vi "Constructor.vi"(7 "TimeZoneInfoId":string, 8 "error in":errorcluster, 9 "ProductFullName":string, 10 "ProductUnitIdentifier":string, 11 "Name":string) -> (0 "error out":errorcluster, 3 "ProductUnit out":refnum<class "ProductUnit.lvclass">)   [LabVIEW 2021, in "ProligentXMLGenerator.lvlib" / "ProductUnit.lvclass"]
uses:
  ProductUnit.lvclass
  ProductUnit.lvclass/ProductUnit.ctl
  Base/DateTime/DateTime.lvclass
  Base/NonEmptyString_50/NonEmptyString_50.lvclass
  Base/FullName/FullName.lvclass
  Data.ctl
  Model/CustomData/CustomData.lvclass
  Base/NonEmptyString_255/NonEmptyString_255.lvclass
  Base/Boolean/Boolean.lvclass
  Model/Document/Document.lvclass
  Model/Characteristic/Characteristic.lvclass
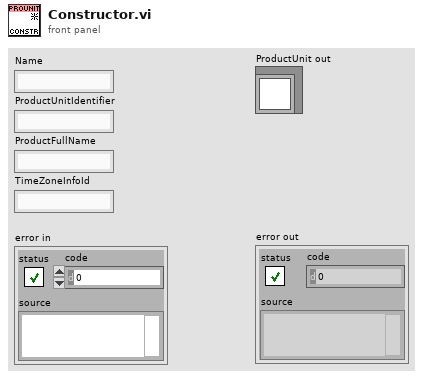
[diagram p1: front panel]
types:
  T1 = typedef "ProligentXMLGenerator.lvlib/ProductUnit.lvclass/Data.ctl" = cluster{"Name":string, "Characteristics":refnum<class "Characteristic.lvclass">[], "Documents":refnum<class "Document.lvclass">[], "CustomData":refnum<class "CustomData.lvclass">, "ProductUnitIdentifier":refnum<class "NonEmptyString_50.lvclass">, "ProductFullName":refnum<class "FullName.lvclass">, "Scrapped":refnum<class "Boolean.lvclass">, "ScrappedTime":refnum<class "DateTime.lvclass">, "CreationTime":refnum<class "DateTime.lvclass">, "ManufacturingTime":refnum<class "DateTime.lvclass">, "ByManufacturer":refnum<class "NonEmptyString_255.lvclass">, "TimeZoneInfoId":string}
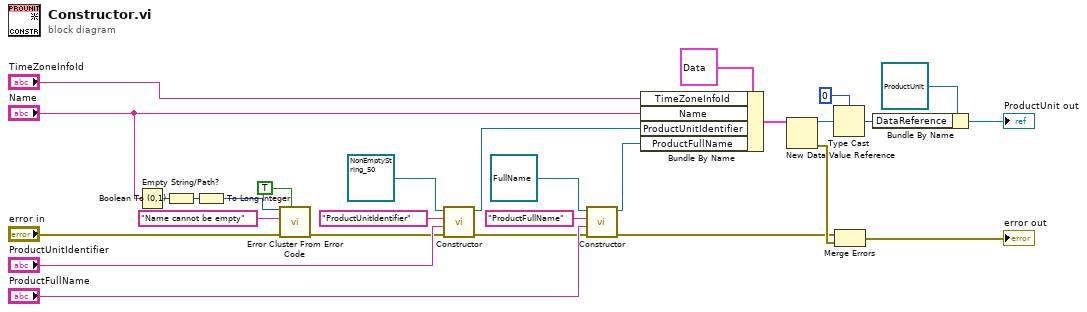
[diagram p0: block diagram]
diagram:
  n1 = Empty String/Path?(string/path="Name") -> (empty?=w16:bool)
  n2 = Boolean To (0,1)(Boolean=w16) -> (0, 1=w15:i16)
  n3 = To Long Integer(number=w15) -> (32bit integer=w14:i32)
  n4 = call <vilib>:"Error Cluster From Error Code.vi"("show call chain? (False)"=TRUE, "error in (no error)"="error in", "error message (\"\")"="Name cannot be empty" ("error message (\"\")"), "error code (0)"=w14) -> ("error out"=w3:errorcluster)  [unwired: 5 in]
  n5 = call-dynamic "Constructor.vi"("error in"=w3, "Value"="ProductUnitIdentifier", "Name"="ProductUnitIdentifier", "String in"=refnum<class "NonEmptyString_50.lvclass"> refnum ("ProligentResultProcessor:NonEmptyString_65")) -> ("error out"=w7:errorcluster, "String out"=w10:refnum<class "NonEmptyString_50.lvclass">)  [unwired: 6 in]
  n6 = call-dynamic "Constructor.vi"("error in"=w7, "Value"="ProductFullName", "Name"="ProductFullName", "String in"=refnum<class "FullName.lvclass"> refnum ("ProligentResultProcessor:NonEmptyString_65")) -> ("error out"=w2:errorcluster, "String out"=w6:refnum<class "FullName.lvclass">)  [unwired: 6 in]
  n7 = Bundle By Name(cluster=T1 {"Name"="", "Characteristics"=[], "Documents"=[], "CustomData"=refnum, "ProductUnitIdentifier"=refnum, "ProductFullName"=refnum, "Scrapped"=refnum, "ScrappedTime"=refnum, "CreationTime"=refnum, "ManufacturingTime"=refnum, "ByManufacturer"=refnum, "TimeZoneInfoId"=""} ("Data"), "TimeZoneInfoId"="TimeZoneInfoId", "Name"="Name", "ProductUnitIdentifier"=w10, "ProductFullName"=w6) -> (w22:T1)
  n8 = New Data Value Reference(data value=w22) -> (data value reference=w21:refnum<data-value>, error out=w18:errorcluster)  [unwired: 1 in]
  n9 = Type Cast(type=u64 0, x=w21) -> (*(type *) &x=w19:u64)
  n10 = Merge Errors(w2, w18) -> (→"error out":errorcluster)
  n11 = Bundle By Name(cluster=refnum<class "ProductUnit.lvclass"> refnum ("ProligentResultProcessor:ProcessRun"), "DataReference"=w19) -> (→"ProductUnit out":refnum<class "ProductUnit.lvclass">)
